vi "ConvertC-D.vi"(3 "Tolerance":dbl, 5 "Distance(mA.)":dbl) -> (0 "LowerDistance(mm.)":dbl format="%#_13g", 1 "NormalDistance(mm.)":dbl, 2 "UpperDistance(mm.)":dbl format="%#_13g")   [LabVIEW 2017]
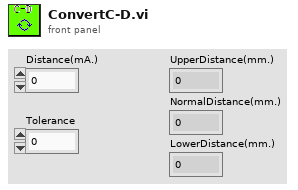
[diagram p1: front panel]
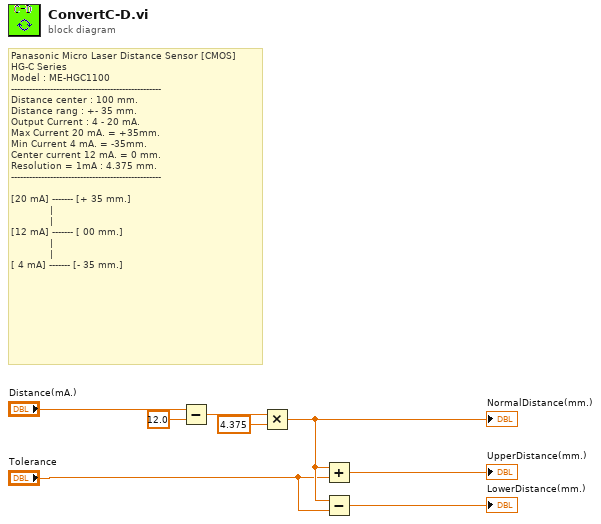
[diagram p0: block diagram]
diagram:
  # "Panasonic Micro Laser Distance Sensor [CMOS]\nHG-C Series \nModel : ME-HGC1100 \n--------------------------------------------------\nDistance center : 100 mm.\nDistance rang : +- 35 mm.\nOutput Current : 4 - 20 mA.\nMax Current 20 mA. = +35mm.\nMin Current 4 mA. = -35mm.\nCenter current 12 mA. = 0 mm.\nResolution = 1mA : 4.375 mm.\n--------------------------------------------------\n\n[20 mA] ------- [+ 35 mm.]\n             |\n             |\n[12 mA] ------- [ 00 mm.]\n             |\n             |\n[ 4 mA] ------- [- 35 mm.]"
  n1 = Subtract(x="Distance(mA.)", y=12.0) -> (x-y=w1:dbl)
  n2 = Multiply(x=w1, y=4.375) -> (x*y=w5:dbl)
  "NormalDistance(mm.)" <- w5
  n3 = Add(x=w5, y="Tolerance") -> (x+y=→"UpperDistance(mm.)":dbl)
  n4 = Subtract(x=w5, y="Tolerance") -> (x-y=→"LowerDistance(mm.)":dbl)
